vi "AMCS_Data.vi"() -> ()   [LabVIEW 2012]
panel:
  in  "AMCS_Profile":i32
  in  "AMCS_Data":u16[][](array[numeric])
  # "AMCS Global Data"
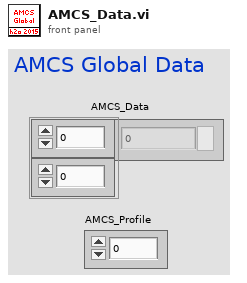
[diagram p1: front panel]
diagram:
